vi "AES Limit APU Speed Request By Acceleration.vi"(10 "APU.Degrees per Tick in":fxp<+/-,47,-4>, 11 "APU.Increment Rate":fxp<+/-,47,-4>) -> (3 "APU.Degrees per Tick out":fxp<+/-,47,-4>)   [LabVIEW 2010, in "AES.lvlib" / "AES FPGA.lvlib"]
doc: "Rate limits the APU speed changes by the APU.Increment Rate value."
uses:
  AES FPGA.lvlib
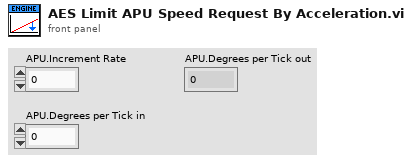
[diagram p1: front panel]
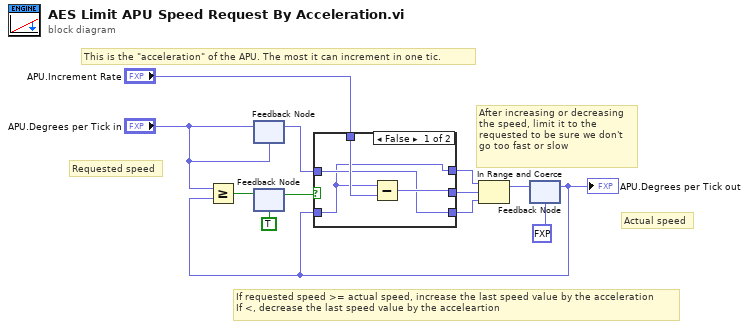
[diagram p0: block diagram]
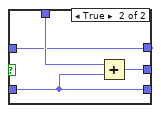
[diagram p2: hidden frame]
diagram:
  # "After increasing or decreasing the speed, limit it to the requested to be sure we don't go too fast or slow"
  # "If requested speed >= actual speed, increase the last speed value by the acceleration\nIf <, decrease the last speed value by the acceleartion"
  # "Actual speed"
  # "Requested speed"
  # "This is the \"acceleration\" of the APU. The most it can increment in one tic."
  n1 = feedback #1("APU.Degrees per Tick in") -> (w12:fxp<+/-,47,-4>)
  n2 = feedback-in #1("APU.Degrees per Tick in") -> ()
  n3 = feedback #2(TRUE) -> (w6:bool)
  n4 = feedback #3(fxp<+/-,47,-4> 0.0 ("APU.Degrees per Tick")) -> (w10:fxp<+/-,47,-4>)
  "APU.Degrees per Tick out" <- w10
  n5 = Greater Or Equal?(x="APU.Degrees per Tick in", y=w10) -> (x >= y?=w5:bool)
  n6 = feedback-in #2(w5) -> ()
  n7 = case shown="False" w6 {
    tunnel: w10 -> [w13 w17]
    tunnel: "APU.Increment Rate" -> [w16 w20]
    tunnel: [w15 w19] -> w8
    tunnel: [w13 w18] -> w3
    tunnel: w12 -> [w14 w18]
    tunnel: [w14 w17] -> w4
    frame False {
      n8 = Subtract(x=w13, y=w16) -> (x-y=w15:fxp<+/-,47,-4>)
    }
    frame True {
      n9 = Add(x=w20, y=w17) -> (x+y=w19:fxp<+/-,47,-4>)
    }
  }
  n10 = In Range and Coerce(upper limit=w3, x=w8, lower limit=w4) -> (coerced(x)=w9:fxp<+/-,47,-4>)  [unwired: 1 out]
  n11 = feedback-in #3(w9) -> ()
